vi "WPI_ADI_IMU_AHRS_RoboBees.vi"(8 "Yaw Axis":enum16{"X", "Y", "Z"}(ring)=enum."Z", 9 "dt (s)":dbl, 10 "IMU Rates":T1) -> (0 "Yaw":dbl(knob) scale=-180.0..180.0, 1 "Roll":dbl(knob) scale=-180.0..180.0, 2 "Pitch":dbl(knob) scale=-90.0..90.0, 3 "Output":dbl[](array[numeric]))   [LabVIEW 2015, in "FRC ADI MXP IMU.lvlib"]
uses:
  FRC ADI MXP IMU.lvlib
panel:
  in  "Tilt Comp (Yaw)":bool
  in  "tau mag":dbl=0.04
  in  "tau acc":dbl=0.6
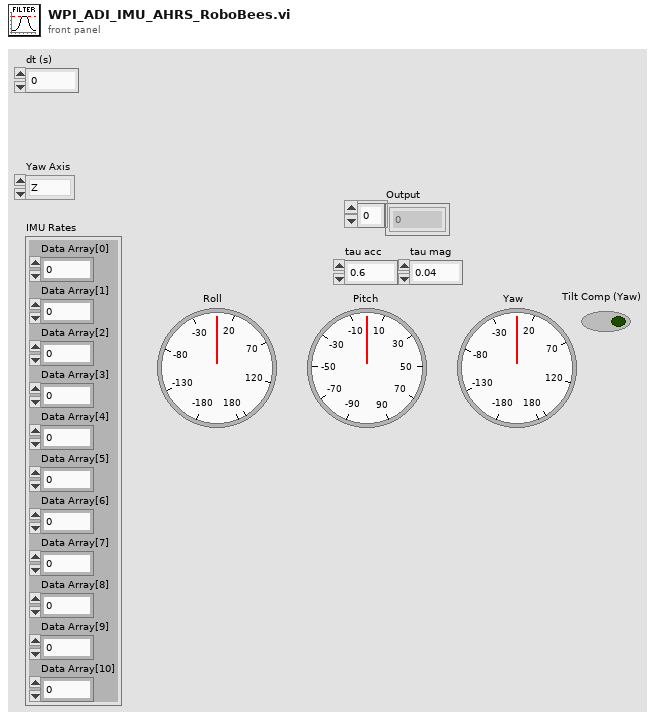
[diagram p1: front panel]
types:
  T1 = cluster{"Data Array[0]":dbl, "Data Array[1]":dbl, "Data Array[2]":dbl, "Data Array[3]":dbl, "Data Array[4]":dbl, "Data Array[5]":dbl, "Data Array[6]":dbl, "Data Array[7]":dbl, "Data Array[8]":dbl, "Data Array[9]":dbl, "Data Array[10]":dbl}
  T2 = cluster{"Xaccel":dbl, "Yaccel":dbl, "Zaccel":dbl}
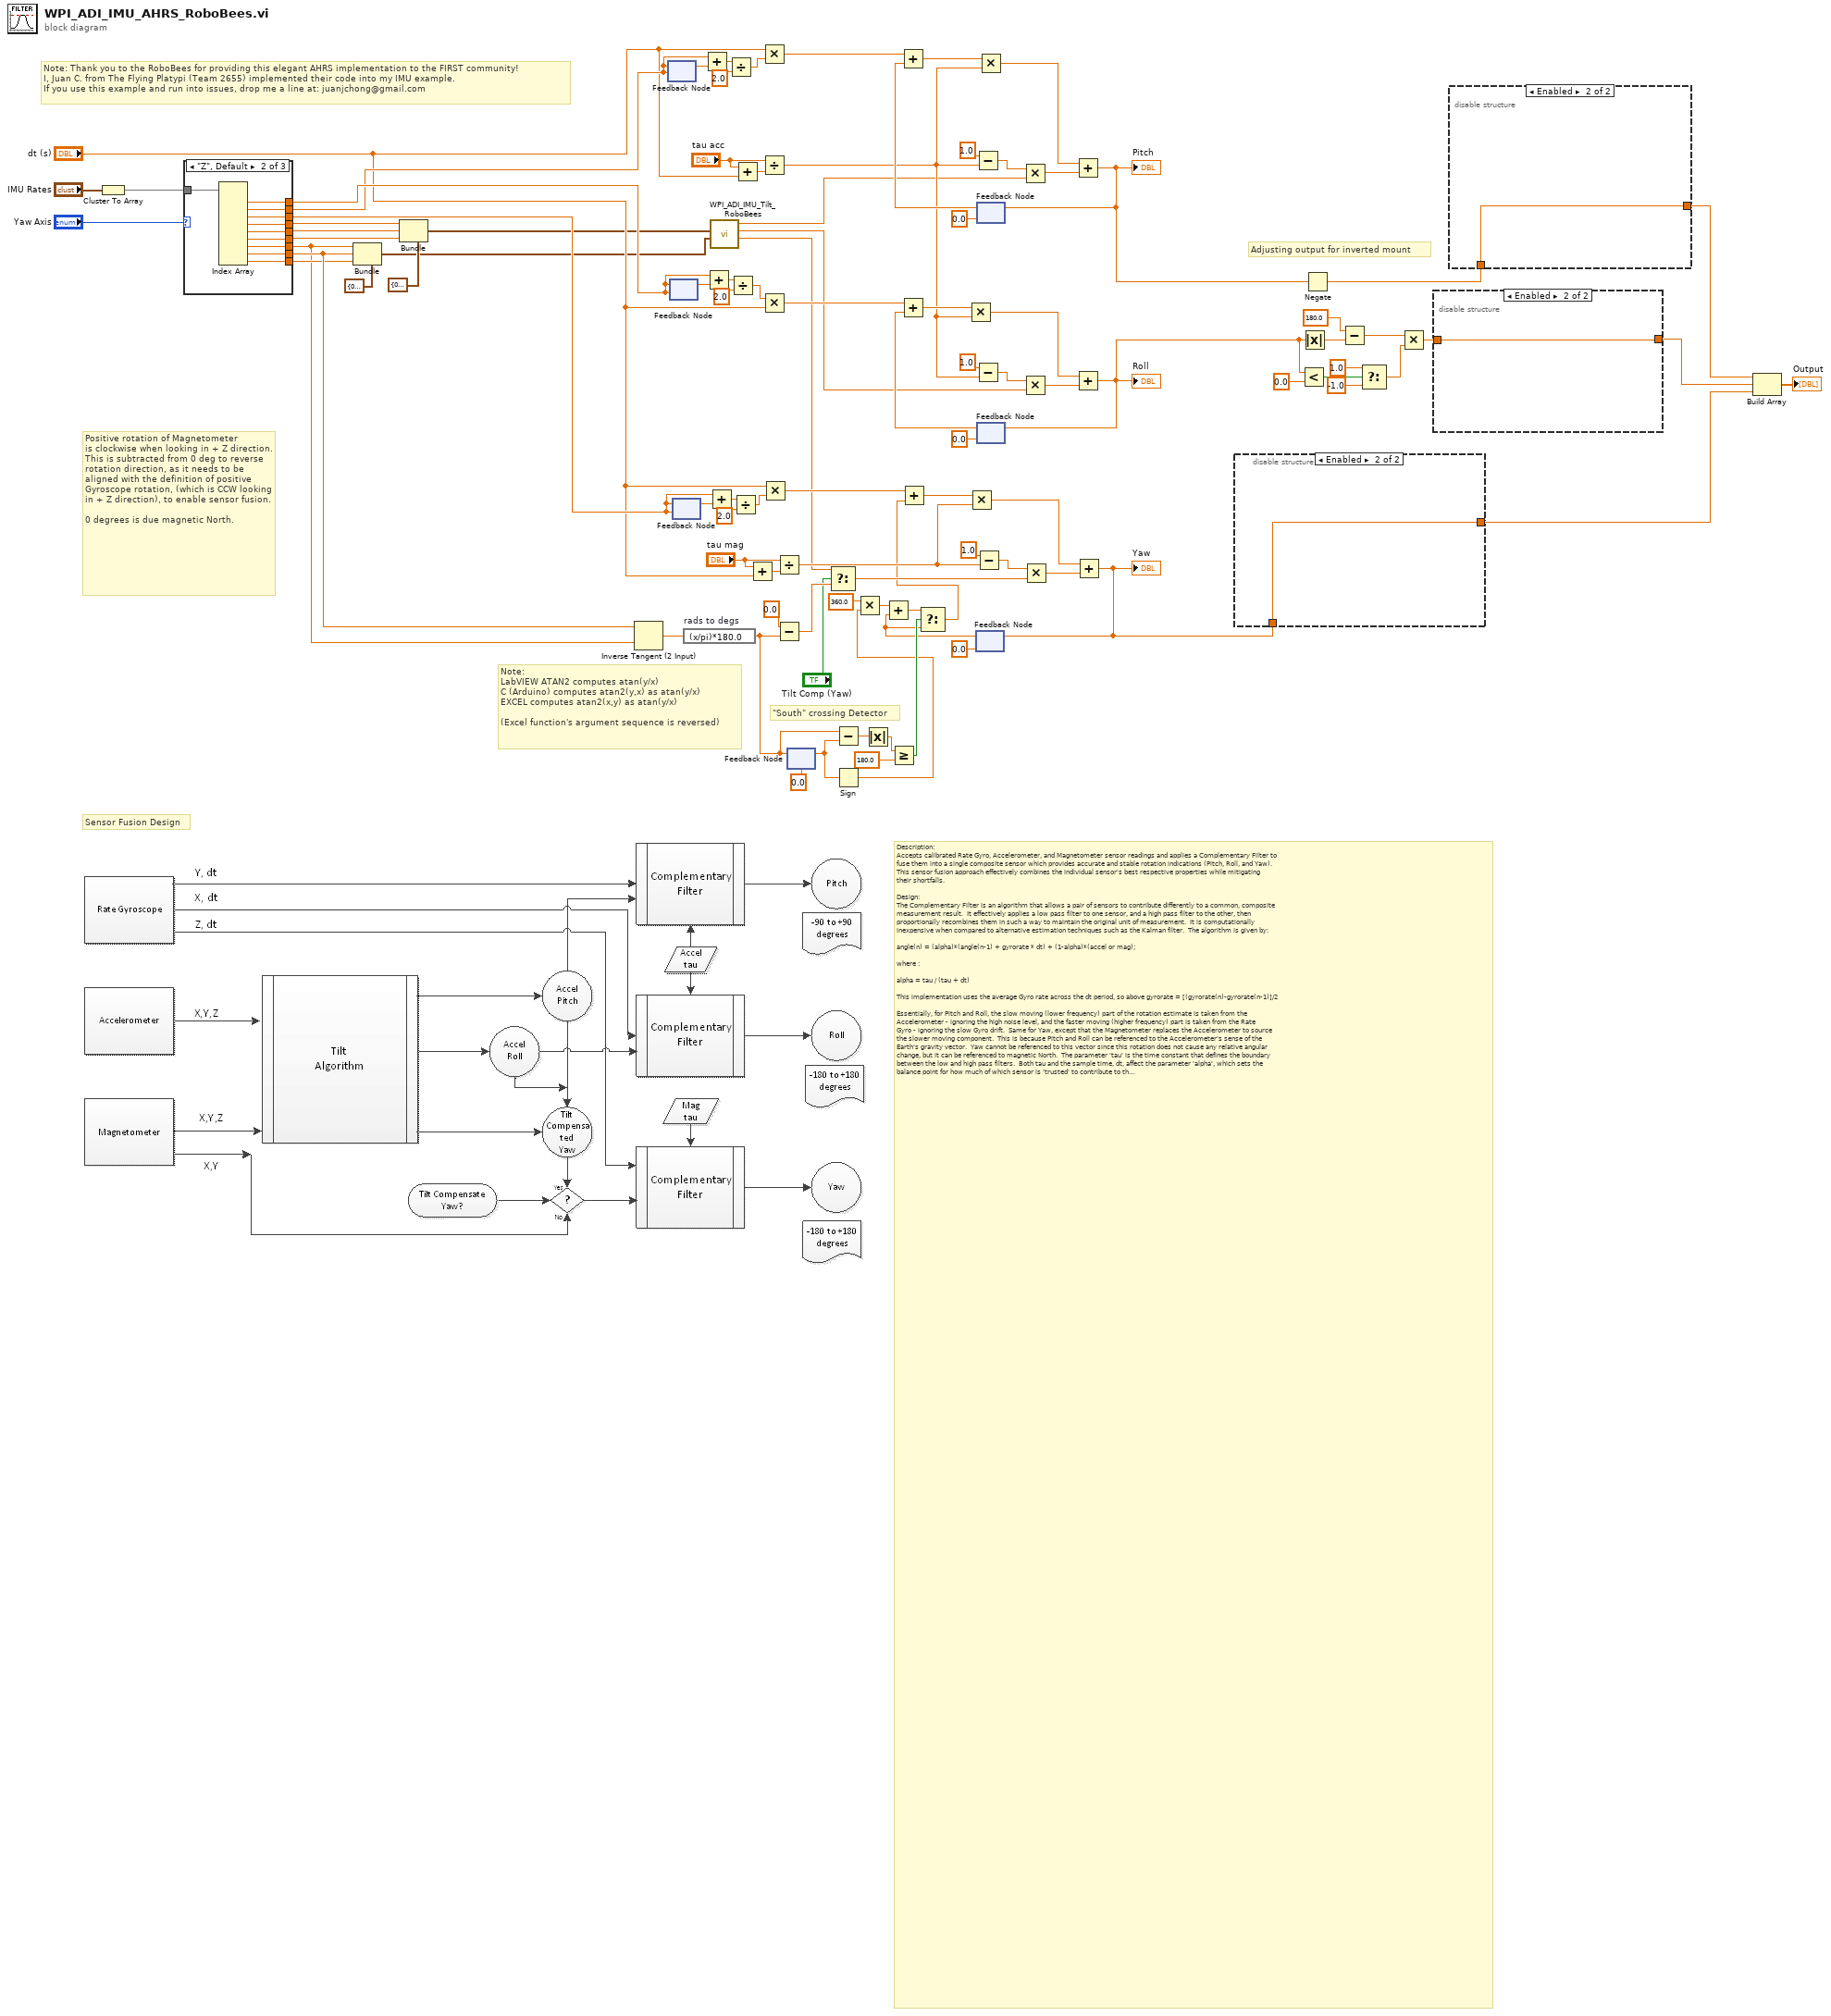
[diagram p0: block diagram]
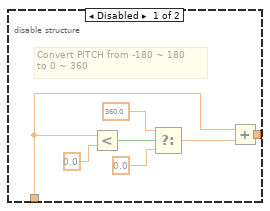
[diagram p2: hidden frame]
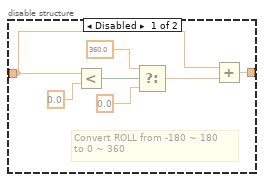
[diagram p3: hidden frame]
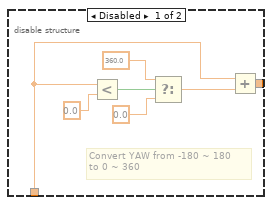
[diagram p4: hidden frame]
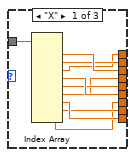
[diagram p5: hidden frame]
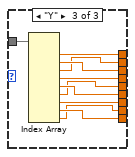
[diagram p6: hidden frame]
diagram:
  # "Note: Thank you to the RoboBees for providing this elegant AHRS implementation to the FIRST community!\nI, Juan C. from The Flying Platypi (Team 2655) implemented their code into my IMU example.\nIf you use this example and run into issues, drop me a line at: juanjchong@gmail.com"
  # "Adjusting output for inverted mount"
  # "Sensor Fusion Design"
  # "Description:\nAccepts calibrated Rate Gyro, Accelerometer, and Magnetometer sensor readings and applies a Complementary Filter to\nfuse them into a single composite sensor which provides accurate and stable rotation indications (Pitch, Roll, and Yaw).\nThis sensor fusion approach effectively combines the individual sensor's best respective properties while mitigating\ntheir shortfalls.\n\nDesign:\nThe Complementary Filter is an algorithm that allows a pair of sensors to contribute differently to a common, composite\nmeasurement result.  It effectively applies a low pass filter to one sensor, and a high pass filter to the other, then\nproportionally recombines them in such a way to maintain the original unit of measurement.  It is computationally\ninexpensive when compared to alternative estimation techniques such as the Kalman filter.  The algorithm is given by:\n\nangle(n) = (alpha)*(angle(n-1) + gyrorate * dt) + (1-alpha)*(accel or mag);\n\nwhere : \n\nalpha = tau / (tau + dt)\n\nThis implementation uses the average Gyro rate across the dt period, so above gyrorate = [(gyrorate(n)-gyrorate(n-1)]/2\n\nEssentially, for Pitch and Roll, the slow moving (lower frequency) part of the rotation estimate is taken from the\nAccelerometer - ignoring the high noise level, and the faster moving (higher frequency) part is taken from the Rate \nGyro - ignoring the slow Gyro drift.  Same for Yaw, except that the Magnetometer replaces the Accelerometer to source\nthe slower moving component.  This is because Pitch and Roll can be referenced to the Accelerometer's sense of the\nEarth's gravity vector.  Yaw cannot be referenced to this vector since this rotation does not cause any relative angular\nchange, but it can be referenced to magnetic North.  The parameter 'tau' is the time constant that defines the boundary\nbetween the low and high pass filters.  Both tau and the sample time, dt, affect the parameter 'alpha', which sets the\nbalance point for how much of which sensor is 'trusted' to contribute to the rotation estimate.\n\nThe Complementary Filter algorithm is applied to each X/Y/Z rotation axis to compute R/P/Y outputs, respectively.\n\nMagnetometer readings are tilt-compensated when Tilt-Comp-(Yaw) is asserted (True), by the IMU TILT subVI.  This\ncreates what is known as a tilt-compensated compass, which allows Yaw to be insensitive to the effects of a\nnon-level sensor, but generates error in Yaw during movement (coordinate acceleration).\n\nThe Yaw \"South\" crossing detector is necessary to allow a smooth transition across the +/- 180 deg discontinuity (inherent\nin the ATAN function).  Since -180 deg is congruent with +180 deg, Yaw needs to jump between these values when\ncrossing South (North is 0 deg).  The design depends upon comparison of successive Yaw readings to detect a cross-over\nevent.  The cross-over detector monitors the current reading and evaluates how far it is from the previous reading.  If it\nis greater than the previous reading by the Discriminant (= 180 deg), then Yaw just crossed South.\n\nBy choosing 180 as the Discriminant, the only way the detector can produce a false positive, assuming a loop iteration\nof 70 msec, is for it to rotate >2,571 dps ... (2,571=180/.07).  This is faster than the ST L3GD20 Gyro can register.  The\ndetector produces a Boolean True upon detecting a South crossing.  This is used to alter the (n-1) Yaw which was\npreviously stored, either adding or subtracting 360 degrees as required to place the previous Yaw in the correct quadrant\nwhenever crossing occurs.  The Modulus function cannot be used here as the Complementary Filter algorithm has 'state'\n(needs to remember previous Yaw).\n \nWe are in effect stitching together two ends of a ruler for 'modular arithmetic' (clock math).\n\nInputs:\nGYRO - Gyro rate and sample time measurements.\nACCEL - Acceleration measurements.\nMAG - Magnetic measurements.\nTAU ACC - tau parameter used to set sensor balance between Accel and Gyro for Roll and Pitch.\nTAU MAG -  tau parameter used to set sensor balance between Mag and Gyro for Yaw.\nTILT COMP (Yaw) - Enables Yaw tilt-compensation if True.\n\nOutputs:\nROLL - Filtered Roll about sensor X-axis.\nPITCH - Filtered Pitch about sensor Y-axis.\nYAW - Filtered Yaw about sensor Z-axis.\n\nVI Properties:\nExecution Reentrancy is set to Non Reentrant Execution\n\nImplementation:\nIt's best to establish the optimum loop sample time first.  See IMU READ implementation notes for guidance.  Each\ntau parameter should then be adjusted to achieve optimum sensor fusion.  tau acc affects Roll and Pitch, tau mag affects\nYaw.  Start at value 1 or 2 and decrease by half each time until the result doesn't drift, but not so far that the result gets\nnoisy.  An optimum tau for this IMU is likely in the range of 1.0 to 0.01, for a loop sample time between 10 and 100 ms.\n\nNote that both sample timing (dt) and tau both affect the balance parameter, 'alpha'.  Adjusting either dt or tau will\nrequire the other to be readjusted to maintain a particular filter performance.\n\nIt is likely best to set Yaw tilt-compensation to off (False) if the Yaw value is to be used as feedback in a closed loop\ncontrol application.  The tradeoff is that Yaw will only be accurate while the robot is level.\n\nSince a Yaw of -180 degrees is congruent with +180 degrees (they represent the same direction), it is possible that the\nYaw output will oscillate between these two values when the sensor happens to be pointing due South, as sensor\nnoise causes slight variation.  You will need to account for this possibility if you are using the Yaw value for decision-\nmaking in code.\n\n----- The RoboBees FRC Team 836! -----  Complement your passion to solve problems with a STEM Education!"
  # "\"South\" crossing Detector"
  # "Positive rotation of Magnetometer\nis clockwise when looking in + Z direction.  This is subtracted from 0 deg to reverse rotation direction, as it needs to be aligned with the definition of positive Gyroscope rotation, (which is CCW looking in + Z direction), to enable sensor fusion.\n\n0 degrees is due magnetic North."
  # "Note:\nLabVIEW ATAN2 computes atan(y/x)\nC (Arduino) computes atan2(y,x) as atan(y/x)\nEXCEL computes atan2(x,y) as atan(y/x)\n\n(Excel function's argument sequence is reversed)"
  n1 = Cluster To Array(cluster="IMU Rates") -> (array=w35:dbl[])
  n2 = case shown="\"Z\", Default" "Yaw Axis" {
    tunnel: [w103 w116 w125] -> w34
    tunnel: [w100 w115 w122] -> w26
    tunnel: w35 -> [w106 w114 w126]
    tunnel: [w97 w113 w119] -> w28
    tunnel: [w101 w112 w120] -> w25
    tunnel: [w102 w111 w121] -> w24
    tunnel: [w104 w110 w123] -> w33
    tunnel: [w105 w109 w124] -> w32
    tunnel: [w98 w108 w117] -> w30
    tunnel: [w99 w107 w118] -> w29
    frame "X" {
      n3 = Index Array(array=w106) -> (element #1=w105:dbl, element #2=w104:dbl, element #3=w103:dbl, element #4=w102:dbl, element #5=w101:dbl, element #6=w100:dbl, element #7=w99:dbl, element #8=w98:dbl, element #9=w97:dbl)  [unwired: 9 in]
    }
    frame "Z", Default {
      n4 = Index Array(array=w114) -> (element #1=w116:dbl, element #2=w110:dbl, element #3=w109:dbl, element #4=w115:dbl, element #5=w112:dbl, element #6=w111:dbl, element #7=w113:dbl, element #8=w108:dbl, element #9=w107:dbl)  [unwired: 9 in]
    }
    frame "Y" {
      n5 = Index Array(array=w126) -> (element #1=w125:dbl, element #2=w124:dbl, element #3=w123:dbl, element #4=w122:dbl, element #5=w121:dbl, element #6=w120:dbl, element #7=w119:dbl, element #8=w118:dbl, element #9=w117:dbl)  [unwired: 9 in]
    }
  }
  n6 = Bundle(cluster=cluster{"Xmag":dbl, "Ymag":dbl, "Zmag":dbl} {"Xmag"=0.0, "Ymag"=0.0, "Zmag"=0.0} ("Mag"), "Xmag"=w28, "Ymag"=w30, "Zmag"=w29) -> (w21:cluster{"Xmag":dbl, "Ymag":dbl, "Zmag":dbl})
  n7 = Bundle(cluster=T2 {"Xaccel"=0.0, "Yaccel"=0.0, "Zaccel"=0.0} ("Accel"), "Xaccel"=w26, "Yaccel"=w25, "Zaccel"=w24) -> (w22:T2)
  n8 = Inverse Tangent (2 Input)(1:w28, 2:w30) -> (0:w69:dbl)
  n9 = feedback #1(w33) -> (w58:dbl)
  n10 = feedback-in #1(w33) -> ()
  n11 = feedback #2(w34) -> (w52:dbl)
  n12 = feedback-in #2(w34) -> ()
  n13 = feedback #3(w32) -> (w50:dbl)
  n14 = feedback-in #3(w32) -> ()
  n15 = expression code="(x/pi)*180.0" "rads to degs"(w69) -> (w39:dbl)
  n16 = Add(x=w33, y=w58) -> (x+y=w57:dbl)
  n17 = Add(x=w34, y=w52) -> (x+y=w53:dbl)
  n18 = Add(x=w32, y=w50) -> (x+y=w49:dbl)
  n19 = call "WPI_ADI_IMU_Tilt_RoboBees.vi"("Mag"=w21, "Accel"=w22) -> ("Yaw"=w18:dbl, "Roll"=w19:dbl, "Pitch"=w20:dbl)  [unwired: 6 in, 1 out]
  n20 = Divide(x=w57, y=2.0) -> (x/y=w55:dbl)
  n21 = Divide(x=w53, y=2.0) -> (x/y=w51:dbl)
  n22 = Divide(x=w49, y=2.0) -> (x/y=w47:dbl)
  n23 = Add(x="tau acc", y="dt (s)") -> (x+y=w95:dbl)
  n24 = Add(x="tau mag", y="dt (s)") -> (x+y=w70:dbl)
  n25 = Multiply(x="dt (s)", y=w55) -> (x*y=w83:dbl)
  n26 = Divide(x="tau acc", y=w95) -> (x/y=w79:dbl)
  n27 = Multiply(x=w51, y="dt (s)") -> (x*y=w93:dbl)
  n28 = Multiply(x="dt (s)", y=w47) -> (x*y=w63:dbl)
  n29 = Divide(x="tau mag", y=w70) -> (x/y=w62:dbl)
  n30 = Subtract(x=0.0 ("y"), y=w39) -> (x-y=w66:dbl)
  n31 = feedback #4(0.0) -> (w40:dbl)
  n32 = feedback-in #4(w39) -> ()
  n33 = Select(t=w18, s="Tilt Comp (Yaw)", f=w66) -> (s? t:f=w67:dbl)
  n34 = Subtract(x=w39, y=w40) -> (x-y=w46:dbl)
  n35 = Sign(1:w40) -> (0:w42:dbl)
  n36 = Multiply(x=360.0 ("y"), y=w42) -> (x*y=w38:dbl)
  n37 = Absolute Value(x=w46) -> (abs(x)=w45:dbl)
  n38 = Greater Or Equal?(x=w45, y=180.0) -> (x >= y?=w43:bool)
  n39 = Subtract(x=1.0, y=w79) -> (x-y=w82:dbl)
  n40 = Subtract(x=1.0, y=w79) -> (x-y=w78:dbl)
  n41 = Subtract(x=1.0, y=w62) -> (x-y=w76:dbl)
  n42 = feedback #5(0.0) -> (w37:dbl)
  n43 = Add(x=w38, y=w37) -> (x+y=w59:dbl)
  n44 = Select(t=w59, s=w43, f=w37) -> (s? t:f=w60:dbl)
  n45 = Add(x=w63, y=w60) -> (x+y=w73:dbl)
  n46 = Multiply(x=w73, y=w62) -> (x*y=w75:dbl)
  n47 = feedback #6(0.0) -> (w87:dbl)
  n48 = Add(x=w83, y=w87) -> (x+y=w84:dbl)
  n49 = Multiply(x=w84, y=w79) -> (x*y=w86:dbl)
  n50 = feedback #7(0.0) -> (w77:dbl)
  n51 = Add(x=w93, y=w77) -> (x+y=w92:dbl)
  n52 = Multiply(x=w92, y=w79) -> (x*y=w90:dbl)
  n53 = Multiply(x=w82, y=w20) -> (x*y=w85:dbl)
  n54 = Multiply(x=w78, y=w19) -> (x*y=w91:dbl)
  n55 = Multiply(x=w76, y=w67) -> (x*y=w74:dbl)
  n56 = Add(x=w86, y=w85) -> (x+y=w8:dbl)
  "Pitch" <- w8
  n57 = feedback-in #6(w8) -> ()
  n58 = Add(x=w90, y=w91) -> (x+y=w7:dbl)
  "Roll" <- w7
  n59 = feedback-in #7(w7) -> ()
  n60 = Add(x=w75, y=w74) -> (x+y=w6:dbl)
  "Yaw" <- w6
  n61 = feedback-in #5(w6) -> ()
  n62 = disable-structure shown="Enabled" {
    disable-tunnel: w6 -> [w128 w134]
    disable-tunnel: [w127 w134] -> w5
    frame Disabled {
      # "Convert YAW from -180 ~ 180 \nto 0 ~ 360"
      n63 = Less?(x=w128, y=0.0) -> (x < y?=w132:bool)
      n64 = Select(t=360.0, s=w132, f=0.0) -> (s? t:f=w129:dbl)
      n65 = Add(x=w128, y=w129) -> (x+y=w127:dbl)
    }
    frame Enabled {
    }
  }
  n66 = Less?(x=w7, y=0.0) -> (x < y?=w13:bool)
  n67 = Absolute Value(x=w7) -> (abs(x)=w16:dbl)
  n68 = Negate(x=w8) -> (-x=w1:dbl)
  n69 = Subtract(x=180.0 ("y"), y=w16) -> (x-y=w10:dbl)
  n70 = Select(t=1.0, s=w13, f=-1.0) -> (s? t:f=w9:dbl)
  n71 = Multiply(x=w10, y=w9) -> (x*y=w4:dbl)
  n72 = disable-structure shown="Enabled" {
    disable-tunnel: w4 -> [w136 w142]
    disable-tunnel: [w135 w142] -> w3
    frame Disabled {
      # "Convert ROLL from -180 ~ 180 \nto 0 ~ 360"
      n73 = Less?(x=w136, y=0.0) -> (x < y?=w140:bool)
      n74 = Select(t=360.0, s=w140, f=0.0) -> (s? t:f=w137:dbl)
      n75 = Add(x=w136, y=w137) -> (x+y=w135:dbl)
    }
    frame Enabled {
    }
  }
  n76 = disable-structure shown="Enabled" {
    disable-tunnel: [w144 w150] -> w2
    disable-tunnel: w1 -> [w143 w150]
    frame Disabled {
      # "Convert PITCH from -180 ~ 180 \nto 0 ~ 360"
      n77 = Less?(x=w143, y=0.0) -> (x < y?=w148:bool)
      n78 = Select(t=360.0, s=w148, f=0.0) -> (s? t:f=w145:dbl)
      n79 = Add(x=w143, y=w145) -> (x+y=w144:dbl)
    }
    frame Enabled {
    }
  }
  n80 = Build Array(w2, w3, w5) -> (→"Output":dbl[])
